vi "Library Save or Load Referenced Controls.vi"(0 "action":enum16{"save", "load"}(ring), 5 "file path":path, 7 "control refs":refnum<vi>[](array[refnum]), 11 "error in (no error)":errorcluster) -> (4 "missing data items? {load}":bool, 6 "file not found? {load}":bool, 8 "dup control refs":refnum<vi>[](array[refnum]), 15 "error out":errorcluster)   [LabVIEW 2012]
doc: "Save or Load the value content of a list of controls (or indicators) as specified through a control reference array. The saved data format consist of an array of clusters containing a string set to the name of the control as well as the variant value of the control. When loading the data, the receiving controls are initialized with the clusters tagged with their name. This allows for storage of any datatype, and makes the procedure instensitive to reordering of the control list. When fewer receiving controls are present than stored data items, no error is generated. When no data item could be matched to one or more receiving controls, a descriptive error is generated. You may wish to ignore this error (flagged by the \"missing data items?\" output) as it might be induced after an intended extension of the receiving set of controls."
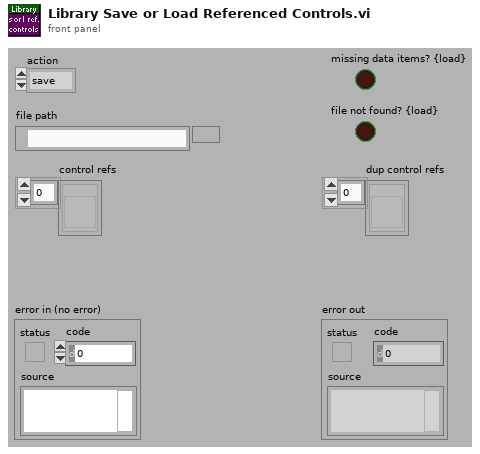
[diagram p1: front panel]
types:
  T1 = enum16{"deny read/write", "deny write-only", "deny none"}
  T2 = enum16{"read/write", "read-only", "write-only", "write-only (truncate)"}
  T3 = typedef "et_Library Error Code Enum.ctl" = enum32{"No error", "Argument error", "Memory is full", "Out of zone", "End of file", "File already open", "Generic file I/O error", "File not found", "File permission error", "Disk is full", "Duplicate path", "Too many files open", "System feature not enabled", "Resource file not found", "Cannot add resource", "Resource not found", "Image not found", "Image memory error", "Pen does not exist", "Config type invalid", "Config token not found", "Config parse error", "Config memory error", "Bad external code format", "Bad external code offset", "External code not present", "Null window", "Destroy window error", "Null menu", "Print aborted", "Bad print record", "Print driver error", "Windows error during printing", "Memory error during printing", "Print dialog error", "Generic print error", "Invalid device refnum", "Device not found", "Device parameter error", "Device unit error", "Cannot open device", "Device call aborted", "Generic error", "Cancelled by user", "Object ID too low", "Object ID too high", "Object not in heap", "Unknown heap", "Unknown object (invalid DefProc)", "Unknown object (DefProc not in table)", "Message out of range", "Invalid (null) method", "Unknown message", "Manager call not supported", "Bad address", "Network operation in progress", "Network operation timed out", "Connection is busy", "Network attribute not supported", "Network error", "Address in use", "System out of memory", "Connection aborted", "Connection refused", "Not connected", "Already connected", "Connection closed", "Initialization error (interapplication manager)", "Bad occurrence", "Wait on unbound occurrence handler", "Occurrence queue overflow", "Datalog type conflict", "Unused", "Unrecognized type (interapplication manager)", "Memory corrupt", "Failed to make temporary DLL", "Old CIN version", "Drag socket not found", "Failed to load drop-object", "Failed to register OLE object", "Failed to release OLE object", "Format specifier type mismatch", "Unknown format specifier", "Too few format specifiers", "Too many format specifiers", "Scan failed", "Newer CIN version", "Error converting to variant", "Runtime menu error", "Password tampered", "Variant attribute not found", "Incompatible variant data type", "Event data is not available", "Event Store is not present", "Occurrence is not found", "Event Queue is not created", "Event info is not available in the type library", "Refnum passed is NULL", "Error retrieving Class GUID", "Error retrieving CoClass GUID", "Error retrieving TypeLib GUID.", "Bad built application magic bytes.", "Specific driver is different from the specific driver associated with the Logical Name.", "There is no session opened to the class driver.", "Max Error", "MAX - Error with config objects", "MAX - Error loading configuration", "MAX - Group not supported", "Singlecast connections can not send to multicast addresses.", "Multicast connections can not send to singlecast addresses.", "Specified IP address not in multicast address range.", "Attempt to write to read-only multicast connection.", "Attempt to read from write-only multicast connection.", "The buffer used to receive a datagram was smaller than the datagram itself", "Error code not enumerated"}
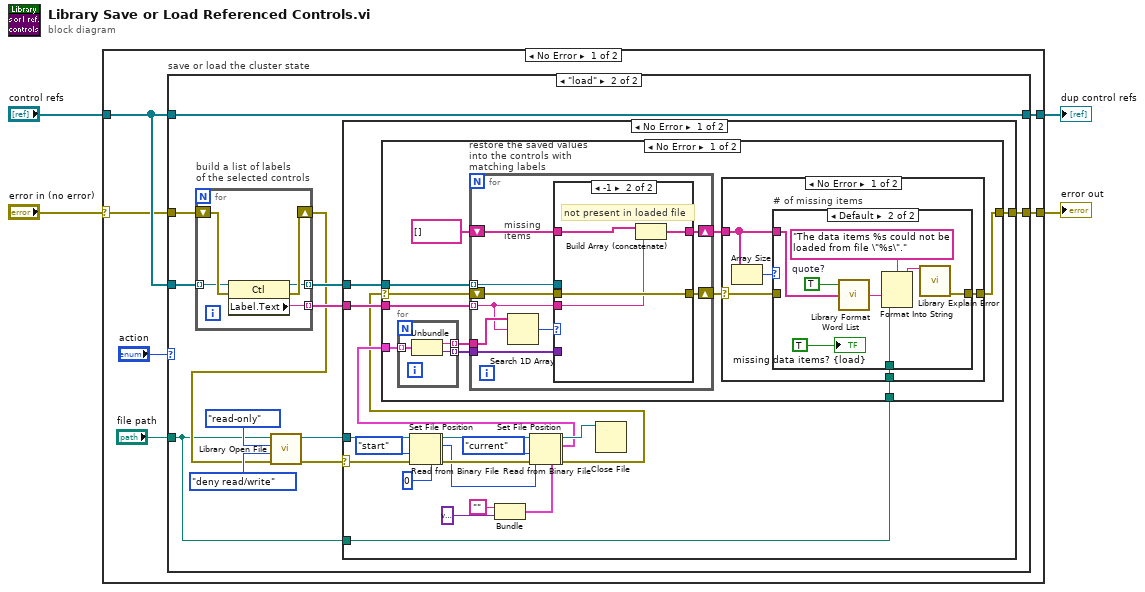
[diagram p0: block diagram]
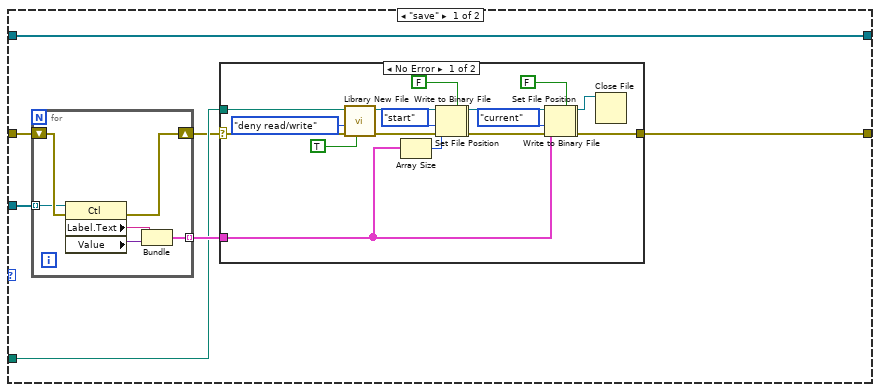
[diagram p2: hidden frame]
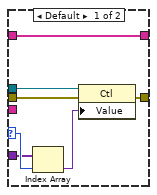
[diagram p6: hidden frame]
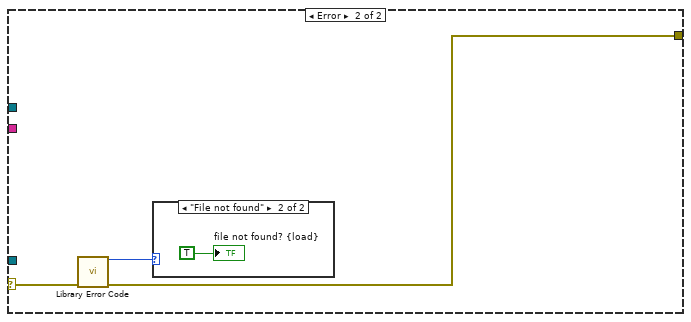
[diagram p8: hidden frame]
diagram:
  n1 = case shown="No Error" "error in (no error)" {
    selector: "error in (no error)" -> [w6 w139]
    tunnel: [w10 w139] -> w4
    tunnel: "control refs" -> [w9 w138]
    tunnel: [w8 w138] -> w2
    frame No Error {
      n2 = case "save or load the cluster state" shown="\"load\"" "action" {
        tunnel: w6 -> [w17 w56]
        tunnel: "file path" -> [w13 w45]
        tunnel: w9 -> [w14 w53]
        tunnel: [w15 w52] -> w8
        tunnel: w9 -> [w15 w52]
        tunnel: [w12 w46] -> w10
        frame "save" {
          n3 = for {
            shift-right: [w43] -> w11
            shift-left: w17 -> [w44]
            tunnel: [w40] -> w16 mode=indexing
            tunnel: w14 -> [w39] mode=indexing
            n4 = property class="Ctl"(reference=w39, error in=w44) -> (error out=w43:errorcluster, "Label.Text"=w42:string, "Value"=w41:variant)  [unwired: 1 out]
            n5 = Bundle("Label.Text"=w42, "Value"=w41) -> (w40:cluster{"Label.Text":string, "Value":variant})  [unwired: 1 in]
          }
          n6 = case shown="No Error" w11 {
            selector: w11 -> [w25 w38]
            tunnel: w16 -> [w31 _]
            tunnel: w13 -> [w27 _]
            tunnel: [w24 w38] -> w12
            frame No Error {
              n7 = call "Library New File.vi"("overwrite (F)"=TRUE, "error in (no error)"=w25, "deny mode (deny none)"=T1."deny read/write" ("deny mode (2)"), "file path"=w27) -> ("error out"=w28:errorcluster, "refnum"=w26:refnum<file>)  [unwired: 6 in]
              n8 = Array Size(array=w31) -> (size(s)=w34:i32)
              n9 = Set File Position(refnum=w26, from (0:start)=enum16{"start", "end", "current"}."start" ("pos mode (0:2)"), error in=w28) -> (refnum out=w23:refnum<file>, error out=w22:errorcluster)  [unwired: 1 in]
              n10 = Write to Binary File(file (use dialog)=w23, data=w34, error in=w22, 5:FALSE ("prepend array or string size? (T)")) -> (refnum out=w33:refnum<file>, error out=w32:errorcluster)  [unwired: 2 in, 1 out]
              n11 = Set File Position(refnum=w33, from (0:start)=enum16{"start", "end", "current"}."current" ("pos mode (0:2)"), error in=w32) -> (refnum out=w20:refnum<file>, error out=w19:errorcluster)  [unwired: 1 in]
              n12 = Write to Binary File(file (use dialog)=w20, data=w31, error in=w19, 5:FALSE ("prepend array or string size? (T)")) -> (refnum out=w36:refnum<file>, error out=w24:errorcluster)  [unwired: 2 in, 1 out]
              n13 = Close File(refnum=w36) -> ()  [unwired: 1 in, 2 out]
            }
            frame Error {
            }
          }
        }
        frame "load" {
          n14 = for "build a list of labels\nof the selected controls" {
            shift-right: [w136] -> w48
            shift-left: w56 -> [w137]
            tunnel: [w135] -> w54 mode=indexing
            tunnel: [w134] -> w55 mode=indexing
            tunnel: w53 -> [w133] mode=indexing
            n15 = property class="Ctl"(reference=w133, error in=w137) -> (reference out=w134:refnum<vi>, error out=w136:errorcluster, "Label.Text"=w135:string)
          }
          n16 = call "Library Open File.vi"("error in (no error)"=w48, "deny mode (deny none)"=T1."deny read/write" ("deny mode (2)"), "open mode (read/write)"=T2."read-only" ("open mode (0)"), "file path"=w45) -> ("error out"=w47:errorcluster, "refnum"=w49:refnum<file>)  [unwired: 2 in]
          n17 = case shown="No Error" w47 {
            selector: w47 -> [w64 w131]
            tunnel: w49 -> [w75 _]
            tunnel: w55 -> [w67 _]
            tunnel: w54 -> [w66 _]
            tunnel: [w63 w130] -> w46
            tunnel: w45 -> [w62 _]
            frame No Error {
              n18 = Set File Position(refnum=w75, from (0:start)=enum16{"start", "end", "current"}."start" ("pos mode (0:2)"), error in=w64) -> (refnum out=w60:refnum<file>, error out=w59:errorcluster)  [unwired: 1 in]
              n19 = Read from Binary File(5:0, 8:w59, 11:w60) -> (0:w73:errorcluster, 2:w71:i32, 3:w74:refnum<file>)  [unwired: 3 in, 1 out]
              n20 = Bundle("", "Value"=variant) -> (w69:cluster{string, "Value":variant})  [unwired: 1 in]
              n21 = Set File Position(refnum=w74, from (0:start)=enum16{"start", "end", "current"}."current" ("pos mode (0:2)"), error in=w73) -> (refnum out=w58:refnum<file>, error out=w57:errorcluster)  [unwired: 1 in]
              n22 = Read from Binary File(5:w69, 8:w57, 10:w71, 11:w58) -> (0:w61:errorcluster, 2:w68:cluster{string, "Value":variant}[], 3:w77:refnum<file>)  [unwired: 2 in, 1 out]
              n23 = case shown="No Error" w61 {
                selector: w61 -> [w88 w128]
                tunnel: w68 -> [w87 _]
                tunnel: w67 -> [w89 _]
                tunnel: w66 -> [w84 _]
                tunnel: [w81 w128] -> w63
                tunnel: w62 -> [w79 _]
                frame No Error {
                  n24 = for {
                    tunnel: w87 -> [w107] mode=indexing
                    tunnel: [w106] -> w86 mode=indexing
                    tunnel: [w105] -> w85 mode=indexing
                    n25 = Unbundle(w107) -> (w106:string, "Value"=w105:variant)
                  }
                  n26 = for "restore the saved values into the controls with matching labels" {
                    tunnel: w89 -> [w115] mode=indexing
                    shift-right: [w114] -> w82
                    shift-left: w88 -> [w113]
                    tunnel: w86 -> [w112]
                    tunnel: w85 -> [w111]
                    tunnel: w84 -> [w110] mode=indexing
                    shift-right: [w109] -> w80
                    shift-left: string[] [] -> [w108]
                    # "missing\nitems"
                    n27 = Search 1D Array(1D array=w112, element=w110) -> (index of element=w116:i32)  [unwired: 1 in]
                    n28 = case shown="-1" w116 {
                      selector: w116 -> [w123 _]
                      tunnel: w115 -> [w118 _]
                      tunnel: w113 -> [w122 w127]
                      tunnel: [w121 w127] -> w114
                      tunnel: w111 -> [w120 _]
                      tunnel: w110 -> [_ w125]
                      tunnel: [w117 w126] -> w109
                      tunnel: w108 -> [w117 w124]
                      frame Default {
                        n29 = Index Array(array=w120, index=w123) -> (element=w119:variant)
                        n30 = property class="Ctl"(reference=w118, error in=w122, "Value"=w119) -> (error out=w121:errorcluster)  [unwired: 1 out]
                      }
                      frame -1 {
                        # "not present in loaded file"
                        n31 = Build Array (concatenate)(w124, w125) -> (w126:string[])
                      }
                    }
                  }
                  n32 = case shown="No Error" w82 {
                    selector: w82 -> [w92 w104]
                    tunnel: [w91 w104] -> w81
                    tunnel: w80 -> [w93 _]
                    tunnel: w79 -> [w90 _]
                    frame No Error {
                      n33 = Array Size(array=w93) -> (size(s)=w94:i32)
                      n34 = case "# of missing items" shown="Default" w94 {
                        tunnel: w93 -> [_ w99]
                        tunnel: w92 -> [w95 _]
                        tunnel: [w95 w103] -> w91
                        tunnel: w90 -> [_ w100]
                        frame 0 {
                        }
                        frame Default {
                          w97 = TRUE  # quote?
                          n35 = call "Library Format Word List.vi"("words"=w99, "quote?"=w97) -> ("formatted list"=w98:string)  [unwired: 3 in]
                          n36 = Format Into String(format string="The data items %s could not be loaded from file \"%s\"." ("Format String"), w98, w100) -> (resulting string=w102:string)  [unwired: 2 in, 1 out]
                          n37 = call "Library Explain Error.vi"("explanation prefix (none)"=w102) -> ("explained error"=w103:errorcluster)  [unwired: 14 in]
                          "missing data items? {load}" <- TRUE
                        }
                      }
                    }
                    frame Error {
                    }
                  }
                }
                frame Error {
                }
              }
              n38 = Close File(refnum=w77) -> ()  [unwired: 1 in, 2 out]
            }
            frame Error {
              n39 = call "Library Error Code.vi"("error"=w131) -> ("error code enum"=w129:T3, "dup error"=w130:errorcluster)  [unwired: 12 in, 1 out]
              n40 = case shown="\"File not found\"" w129 {
                frame Default {
                }
                frame "File not found" {
                  "file not found? {load}" <- TRUE ("file not found? {load}")
                }
              }
            }
          }
        }
      }
    }
    frame Error {
    }
  }
  "error out" <- w4
  "dup control refs" <- w2
